vi "Loop_Vision.vi"() -> ()   [LabVIEW 2017, in "VisionSystem.lvlib"]
uses:
  VisionSystem.lvlib
  ENUM_Vision_State.ctl
  ENUM_Vision_Action.ctl
  Cluster_Results.ctl
  Cluster_Targeting Data.ctl
  Cluster_SGL Point.ctl
  Cluster_UI DBL Box.ctl
  Cluster_Vision Status.ctl
  Enum_ Field Targets.ctl
  Cluster_HW_Status.ctl
  <vilib>/vision/Image Controls.llb/IMAQ Image.ctl
  TypeDefs/Cluster_Camera Settings.ctl
  <vilib>/Rock Robotics/WPI/Camera/WPI_CameraImageSize.ctl
  <vilib>/Rock Robotics/WPI/Camera/WPI_CameraFrameRate.ctl
  <vilib>/Rock Robotics/WPI/Camera/WPI_CameraWhite Balance Values.ctl
  <vilib>/Rock Robotics/WPI/Camera/WPI_CameraExposure Values.ctl
  <vilib>/Rock Robotics/WPI/Camera/WPI_CameraDevRef.ctl
  Cluster_Vision Settings.ctl
  Cluster_Threshold Settings.ctl
  Cluster_Line.ctl
  ENUM_Camera Types.ctl
  _SHARE ALL/Global Share All/Global_STOP.vi
  Global_HW Status.vi
  Global_Vision Status.vi
panel:
  in  "Tab":enum32{"Boiler Settings", "Peg Settings"}(tab)
  in  "Boiler Setting":T1={"Color"={"Hue"={230.0, 10.0}, "Sat"={60.71428571428572, 255.0}, "Val"={63.75000000000001, 215.53571428571428}}, "Particles"=10.0, "Score Cutoff"=50.0, "Line Border"={"Top"=6.0, "Bottom"=1.0}, "Size Limit %"=0.04} {"Color"."Hue" scale=0.0..255.0 scale format="%#_3g"}
  in  "Peg Settings":T1={"Color"={"Hue"={235.0, 13.0}, "Sat"={0.0, 255.0}, "Val"={88.03571428571429, 221.60714285714286}}, "Particles"=10.0, "Score Cutoff"=50.0, "Line Border"={"Top"=6.0, "Bottom"=1.0}, "Size Limit %"=0.04} {"Color"."Hue" scale=0.0..255.0 scale format="%#_3g"}
  in  "Show Images":bool
  out "Errors":errorcluster[](array[cluster])
  out "HW_Vison_Status":T3 {"Cam Setings"."Saturation" min=0 max=100 step=1; "Cam Setings"."Sharpness" min=0 max=100 step=1; "Cam Setings"."Brightness" min=0 max=100 step=1; "Cam Setings"."Exposure (%)" min=0.0 max=100.0 step=1.0}
  out "Target":T10
  in  "Restore Settings":bool
  in  "Save Settings":bool
  out "Qualified Particles":i32
  out "Vision Status":T12
  out "Results":T13 {"Score" format="%#_3g"; "Pixels"."Box"."Bottom" format="%#_3g"; "Pixels"."Box"."Right" format="%#_3g"; "Pixels"."Box"."Top" format="%#_3g"; "Pixels"."Box"."Left" format="%#_3g"; "Normalized"."Box"."Bottom" format="%#_3g"; "Normalized"."Box"."Right" format="%#_3g"; "Normalized"."Box"."Top" format="%#_3g"; "Normalized"."Box"."Left" format="%#_3g"; "Distance (ft)" format="%#_3g"}
  out "cycle time":dbl
  out "Camera":T4(plugin-control)
  out "Mask":T4(plugin-control)
  out "Action":T17
  out "Current State":T18
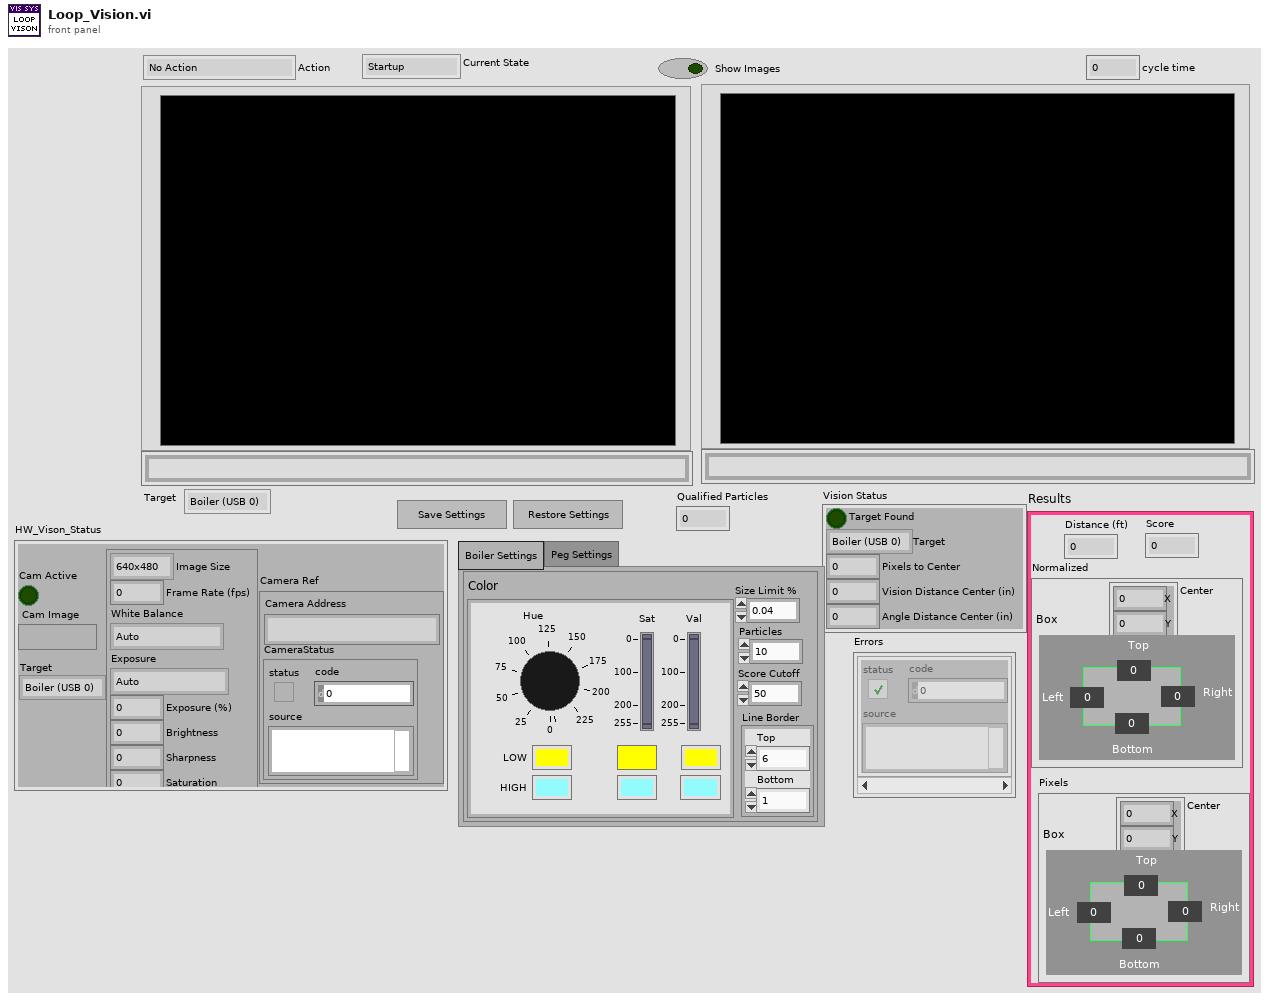
[diagram p1: front panel]
types:
  T1 = typedef "VisionSystem.lvlib/Cluster_Vision Settings.ctl" = cluster{"Color":T2, "Particles":dbl, "Score Cutoff":dbl, "Line Border":cluster{"Top":dbl, "Bottom":dbl}, "Size Limit %":dbl}
  T2 = typedef "VisionSystem.lvlib/Cluster_Threshold Settings.ctl" = cluster{"Hue":cluster{dbl, dbl}, "Sat":cluster{dbl, dbl}, "Val":cluster{dbl, dbl}}
  T3 = typedef "VisionSystem.lvlib/Cluster_HW_Status.ctl" = cluster{"Cam Active":bool, "Cam Image":T4, "Cam Setings":T5, "Target":T10, "Camera Ref":T11}
  T4 = typedef "IMAQ Image.ctl" = refnum<image>
  T5 = typedef "Cluster_Camera Settings.ctl" = cluster{"Image Size":T6, "Frame Rate (fps)":T7, "White Balance":T8, "Exposure":T9, "Exposure (%)":dbl, "Brightness":i32, "Sharpness":i32, "Saturation":i32}
  T6 = typedef "WPI_CameraImageSize.ctl" = enum16{"640x480", "320x240", "160x120", "Custom"}
  T7 = typedef "WPI_CameraFrameRate.ctl" = u32
  T8 = typedef "WPI_CameraWhite Balance Values.ctl" = enum16{"Auto", "Fixed indoor", "Fixed outdoor 1", "Fixed outdoor 2", "Fixed fluorescent 1", "Fixed fluorescent 2", "Hold current", "Custom"}
  T9 = typedef "WPI_CameraExposure Values.ctl" = enum16{"Auto", "Flicker-free 50 Hz", "Flicker-free 60 Hz", "Hold current", "Custom"}
  T10 = typedef "VisionSystem.lvlib/Enum_ Field Targets.ctl" = enum16{"Boiler (USB 0)", "Rope (USB 1)"}
  T11 = typedef "WPI_CameraDevRef.ctl" = cluster{"Camera Address":string, "CameraStatus":errorcluster}
  T12 = typedef "VisionSystem.lvlib/Cluster_Vision Status.ctl" = cluster{"Target Found":bool, "Target":T10, "Pixels to Center":dbl, "Vision Distance Center (in)":dbl, "Angle Distance Center (in)":dbl}
  T13 = typedef "VisionSystem.lvlib/Cluster_Results.ctl" = cluster{"Distance (ft)":dbl, "Score":dbl, "Normalized":T14, "Pixels":T14}
  T14 = typedef "VisionSystem.lvlib/Cluster_Targeting Data.ctl" = cluster{"Center":T15, "Box":T16}
  T15 = typedef "VisionSystem.lvlib/Cluster_SGL Point.ctl" = cluster{"X":sgl, "Y":sgl}
  T16 = typedef "VisionSystem.lvlib/Cluster_UI DBL Box.ctl" = cluster{"Left":dbl, "Top":dbl, "Right":dbl, "Bottom":dbl}
  T17 = typedef "VisionSystem.lvlib/ENUM_Vision_Action.ctl" = enum16{"No Action", "Reset Time", "Open Mask", "Close Mask", "Save Settings to File", "Restore Settings from File", "Build Mask", "Analyze Particles", "Cull and Group", "Calculate Distance", "Build Results", "Label Image"}
  T18 = typedef "VisionSystem.lvlib/ENUM_Vision_State.ctl" = enum16{"Startup", "Idle", "Analyze", "Shutdown"}
  T19 = typedef "VisionSystem.lvlib/Cluster_Line.ctl" = cluster{"Left":dbl, "Top":dbl, "Right":dbl, "Bottom":dbl}
  T20 = typedef "Particle Parameters" = i32
  T21 = cluster{"Actions":T17[], "State":T18, "Current Time":timestamp, "Start Time":timestamp, "Loop Time (ms)":u32, "HW_Status":T3, "Vision Status_OUT":T12, "Tab":enum32{"Boiler Settings", "Peg Settings"}, "Peg Settings":T1, "Boiler Settings":T1, "Mask":T4, "Measure List":T20[], "Current Settings":T1, "Show Images":bool, "Sorted Data":dbl[][], "Particles":i32, "Image":T4, "Center Out":T15, "Score Out":dbl, "Line Out":T19, "Rect Out":T16, "Distance (ft)":dbl, "Edges":T15[], "Results Out":T13, "Actions List":T17[]}
  T22 = typedef "VisionSystem.lvlib/ENUM_Camera Types.ctl" = enum16{"206", "1011", "1013", "MS HD3000 square", "MS HD3000 640x480"}
  T23 = typedef "Image Type" = u32
  T24 = typedef "VisionSystem.lvlib/Cluster_DBL Point.ctl" = cluster{"X":dbl, "Y":dbl}
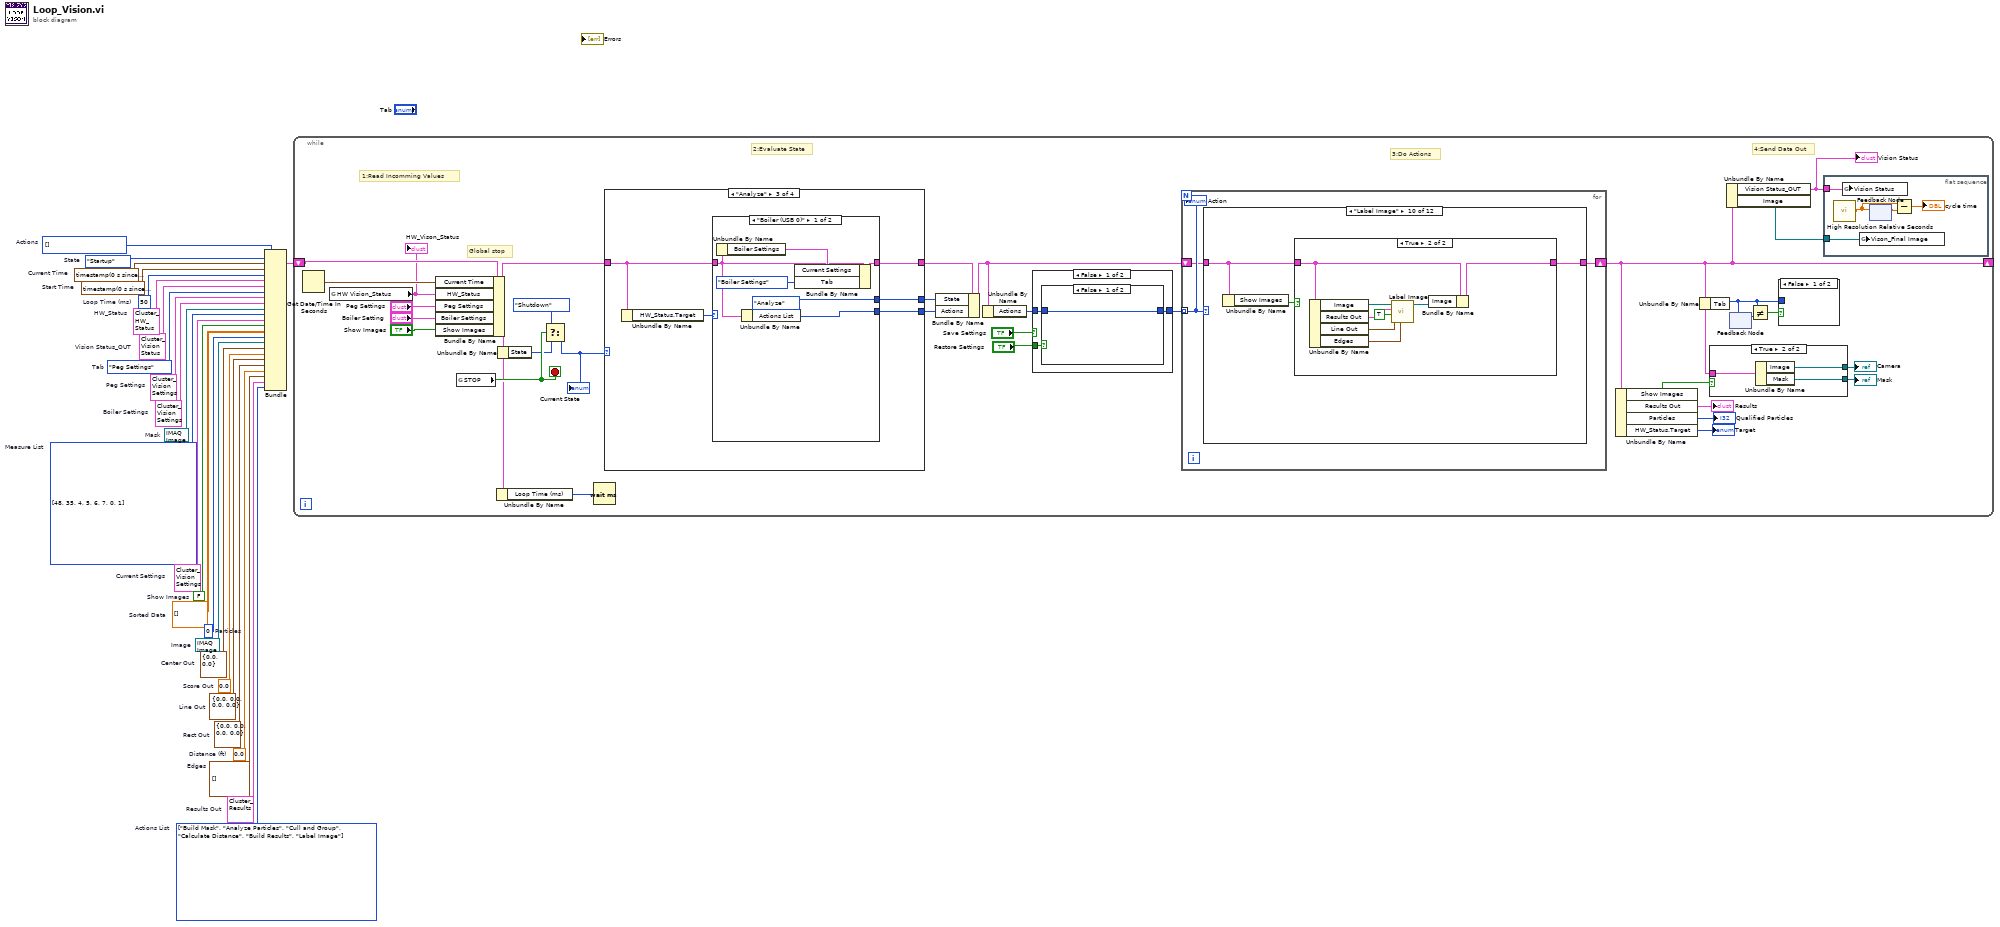
[diagram p0: block diagram]
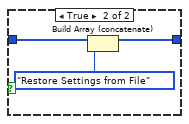
[diagram p2: hidden frame]
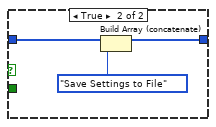
[diagram p3: hidden frame]
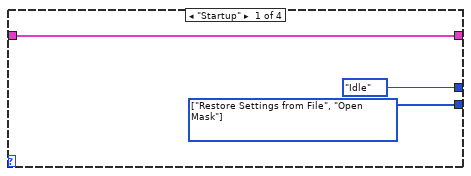
[diagram p4: hidden frame]
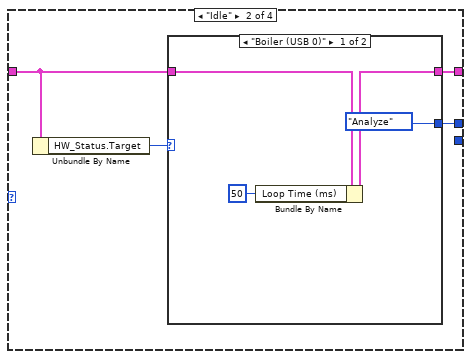
[diagram p5: hidden frame]
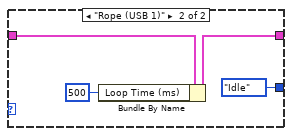
[diagram p6: hidden frame]
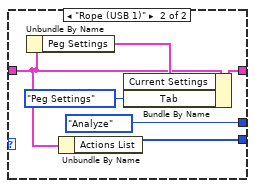
[diagram p7: hidden frame]
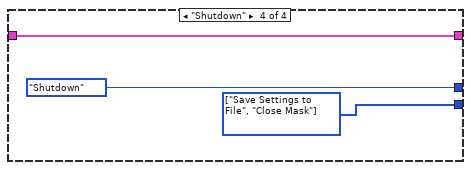
[diagram p8: hidden frame]
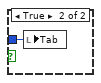
[diagram p10: hidden frame]
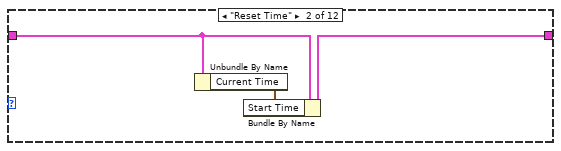
[diagram p12: hidden frame]
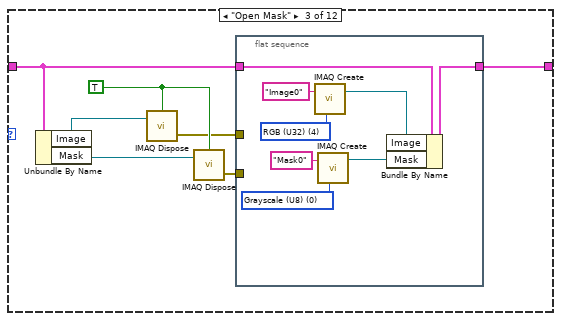
[diagram p13: hidden frame]
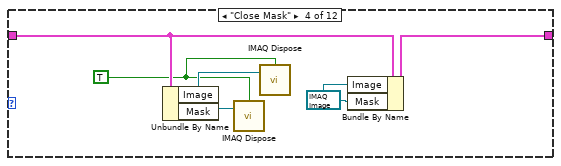
[diagram p14: hidden frame]
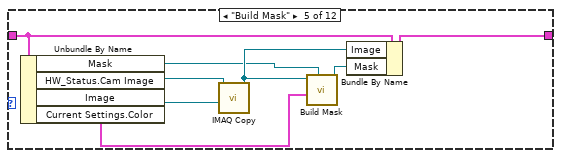
[diagram p15: hidden frame]
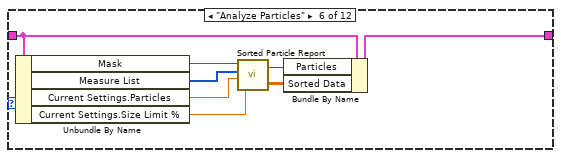
[diagram p16: hidden frame]
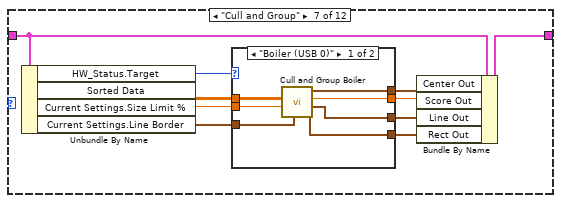
[diagram p17: hidden frame]
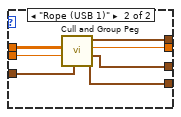
[diagram p18: hidden frame]
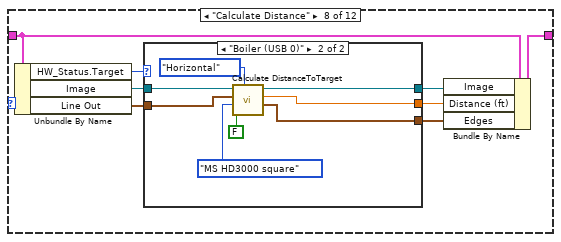
[diagram p19: hidden frame]
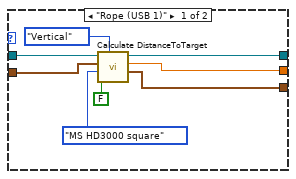
[diagram p20: hidden frame]
diagram:
  w1 = T17[] [enum."Build Mask", enum."Analyze Particles", enum."Cull and Group", enum."Calculate Distance", enum."Build Results", enum."Label Image"] items=["No Action", "Reset Time", "Open Mask", "Close Mask", "Save Settings to File", "Restore Settings from File", "Build Mask", "Analyze Particles", "Cull and Group", "Calculate Distance", "Build Results", "Label Image"]  # Actions List
  w2 = T13 {"Distance (ft)"=0.0, "Score"=0.0, "Normalized"={"Center"={"X"=0.0, "Y"=0.0}, "Box"={"Left"=0.0, "Top"=0.0, "Right"=0.0, "Bottom"=0.0}}, "Pixels"={"Center"={"X"=0.0, "Y"=0.0}, "Box"={"Left"=0.0, "Top"=0.0, "Right"=0.0, "Bottom"=0.0}}}  # Results Out
  w3 = T15[] []  # Edges
  w4 = 0.0  # Distance (ft)
  w5 = T16 {"Left"=0.0, "Top"=0.0, "Right"=0.0, "Bottom"=0.0}  # Rect Out
  w6 = T19 {"Left"=0.0, "Top"=0.0, "Right"=0.0, "Bottom"=0.0}  # Line Out
  w7 = 0.0  # Score Out
  w8 = T15 {"X"=0.0, "Y"=0.0}  # Center Out
  w9 = T4 refnum  # Image
  w10 = 0  # Particles
  w11 = dbl[][] []  # Sorted Data
  w12 = FALSE  # Show Images
  w13 = T1 {"Color"={"Hue"={235.0, 13.0}, "Sat"={97.0, 224.64285714285714}, "Val"={170.0, 255.0}}, "Particles"=10.0, "Score Cutoff"=50.0, "Line Border"={"Top"=6.0, "Bottom"=1.0}, "Size Limit %"=0.04}  # Current Settings
  w14 = T20[] [48, 35, 4, 5, 6, 7, 0, 1] items=["Center of Mass X", "Center of Mass Y", "First Pixel X", "First Pixel Y", "Bounding Rect Left", "Bounding Rect Top", "Bounding Rect Right", "Bounding Rect Bottom", "Max Feret Diameter Start X", "Max Feret Diameter Start Y", "Max Feret Diameter End X", "Max Feret Diameter End Y", "Max Horiz. Segment Length Left", "Max Horiz. Segment Length Right", "Max Horiz. Segment Length Row", "-", "Bounding Rect Width", "Bounding Rect Height", "Bounding Rect Diagonal", "Perimeter", "Convex Hull Perimeter", "Holes' Perimeter", "Max Feret Diameter", "Equivalent Ellipse Major Axis", "Equivalent Ellipse Minor Axis", "Equivalent Ellipse Minor Axis (Feret)", "Equivalent Rect Long Side", "Equivalent Rect Short Side", "Equivalent Rect Diagonal", "Equivalent Rect Short Side (Feret)", "Average Horiz. Segment Length", "Average Vert. Segment Length", "Hydraulic Radius", "Waddel Disk Diameter", "-", "Area", "Holes' Area", "Particle & Holes' Area", "Convex Hull Area", "Image Area", "-", "Number of Holes", "Number of Horiz. Segments", "Number of Vert. Segments", "-", "Orientation", "Max Feret Diameter Orientation", "-", "% Area/Image Area", "% Area/(Particle & Holes' Area)", "Ratio of Equivalent Ellipse Axes", "Ratio of Equivalent Rect Sides", "-", "Elongation Factor", "Compactness Factor", "Heywood Circularity Factor", "Type Factor", "-", "Sum X", "Sum Y", "Sum XX", "Sum XY", "Sum YY", "Sum XXX", "Sum XXY", "Sum XYY", "Sum YYY", "-", "Moment of Inertia XX", "Moment of Inertia XY", "Moment of Inertia YY", "Moment of Inertia XXX", "Moment of Inertia XXY", "Moment of Inertia XYY", "Moment of Inertia YYY", "Norm. Moment of Inertia XX", "Norm. Moment of Inertia XY", "Norm. Moment of Inertia YY", "Norm. Moment of Inertia XXX", "Norm. Moment of Inertia XXY", "Norm. Moment of Inertia XYY", "Norm. Moment of Inertia YYY", "Hu Moment 1", "Hu Moment 2", "Hu Moment 3", "Hu Moment 4", "Hu Moment 5", "Hu Moment 6", "Hu Moment 7"]  # Measure List
  w15 = T4 refnum  # Mask
  w16 = T1 {"Color"={"Hue"={235.0, 13.0}, "Sat"={97.0, 224.64285714285714}, "Val"={170.0, 255.0}}, "Particles"=10.0, "Score Cutoff"=50.0, "Line Border"={"Top"=6.0, "Bottom"=1.0}, "Size Limit %"=0.04}  # Boiler Settings
  w17 = T1 {"Color"={"Hue"={235.0, 13.0}, "Sat"={97.0, 224.64285714285714}, "Val"={170.0, 255.0}}, "Particles"=10.0, "Score Cutoff"=50.0, "Line Border"={"Top"=6.0, "Bottom"=1.0}, "Size Limit %"=0.04}  # Peg Settings
  w18 = enum32{"Boiler Settings", "Peg Settings"}."Peg Settings"  # Tab
  w19 = T12 {"Target Found"=FALSE, "Target"=enum."Boiler (USB 0)", "Pixels to Center"=0.0, "Vision Distance Center (in)"=0.0, "Angle Distance Center (in)"=0.0}  # Vision Status_OUT
  w20 = T3 {"Cam Active"=FALSE, "Cam Image"=refnum, "Cam Setings"={"Image Size"=enum."640x480", "Frame Rate (fps)"=0, "White Balance"=enum."Auto", "Exposure"=enum."Auto", "Exposure (%)"=0.0, "Brightness"=0, "Sharpness"=0, "Saturation"=0}, "Target"=enum."Boiler (USB 0)", "Camera Ref"={"Camera Address"="", "CameraStatus"={"status"=FALSE, "code"=0, "source"=""}}}  # HW_Status
  w21 = u32 50  # Loop Time (ms)
  w22 = T17[] [] items=["No Action", "Reset Time", "Open Mask", "Close Mask", "Save Settings to File", "Restore Settings from File", "Build Mask", "Analyze Particles", "Cull and Group", "Calculate Distance", "Build Results", "Label Image"]  # Actions
  w23 = timestamp(0 s since 1904-01-01)  # Start Time
  w24 = timestamp(0 s since 1904-01-01)  # Current Time
  w25 = ENUM_Vision_State."Startup"  # State
  n1 = Bundle("Actions"=w22, "State"=w25, "Current Time"=w24, "Start Time"=w23, "Loop Time (ms)"=w21, "HW_Status"=w20, "Vision Status_OUT"=w19, "Tab"=w18, "Peg Settings"=w17, "Boiler Settings"=w16, "Mask"=w15, "Measure List"=w14, "Current Settings"=w13, "Show Images"=w12, "Sorted Data"=w11, "Particles"=w10, "Image"=w9, "Center Out"=w8, "Score Out"=w7, "Line Out"=w6, "Rect Out"=w5, "Distance (ft)"=w4, "Edges"=w3, "Results Out"=w2, "Actions List"=w1) -> (w26:T21)  [unwired: 1 in]
  n2 = while {
    shift-right: [w32] -> _
    shift-left: w26 -> [w58]
    stop <- w53 stop-if-true
    # "1:Read Incomming Values"
    # "2:Evaluate State"
    # "3:Do Actions"
    # "4:Send Data Out"
    # "Global stop"
    n3 = Get Date/Time In Seconds() -> (seconds since 1Jan1904=w57:timestamp)
    n4 = global read "Global_HW Status.vi" "HW Vision_Status"() -> (w39:T3)
    "HW_Vison_Status" <- w39
    n5 = Bundle By Name(cluster=w58, "Current Time"=w57, "HW_Status"=w39, "Peg Settings"="Peg Settings", "Boiler Settings"="Boiler Setting", "Show Images"="Show Images") -> (w48:T21)
    n6 = global read "Global_STOP.vi" "STOP"() -> (w53:bool)
    n7 = Unbundle By Name(w48) -> ("Loop Time (ms)"=w49:u32)
    n8 = Unbundle By Name(w48) -> ("State"=w51:T18)
    n9 = Select(t=ENUM_Vision_State."Shutdown" ("State"), s=w53, f=w51) -> (s? t:f=w50:T18)
    "Current State" <- w50
    n10 = Wait (ms)(milliseconds to wait=w49) -> ()  [unwired: 1 out]
    n11 = case shown="\"Analyze\"" w50 {
      tunnel: w48 -> [w76 w79 w92 w108]
      tunnel: [w76 w78 w91 w108] -> w56
      tunnel: [ENUM_Vision_State."Idle" ("State") w77 w90 ENUM_Vision_State."Shutdown" ("State")] -> w55
      tunnel: [w75 _ w89 w106] -> w54
      frame "Startup" {
        w75 = T17[] [enum."Restore Settings from File", enum."Open Mask"] items=["No Action", "Reset Time", "Open Mask", "Close Mask", "Save Settings to File", "Restore Settings from File", "Build Mask", "Analyze Particles", "Cull and Group", "Calculate Distance", "Build Results", "Label Image"] ("Actions")
      }
      frame "Idle" {
        n12 = Unbundle By Name(w79) -> ("HW_Status.Target"=w80:T10)
        n13 = case shown="\"Boiler (USB 0)\"" w80 {
          tunnel: w79 -> [w83 w87]
          tunnel: [w82 w86] -> w78
          tunnel: [ENUM_Vision_State."Analyze" ("State") ENUM_Vision_State."Idle" ("State")] -> w77
          frame "Boiler (USB 0)" {
            n14 = Bundle By Name(cluster=w83, "Loop Time (ms)"=u32 50) -> (w82:T21)
          }
          frame "Rope (USB 1)" {
            n15 = Bundle By Name(cluster=w87, "Loop Time (ms)"=u32 500) -> (w86:T21)
          }
        }
      }
      frame "Analyze" {
        n16 = Unbundle By Name(w92) -> ("HW_Status.Target"=w93:T10)
        n17 = case shown="\"Boiler (USB 0)\"" w93 {
          tunnel: w92 -> [w95 w101]
          tunnel: [w98 w104] -> w91
          tunnel: [ENUM_Vision_State."Analyze" ("State") ENUM_Vision_State."Analyze" ("State")] -> w90
          tunnel: [w94 w100] -> w89
          frame "Boiler (USB 0)" {
            n18 = Unbundle By Name(w95) -> ("Boiler Settings"=w96:T1)
            n19 = Unbundle By Name(w95) -> ("Actions List"=w94:T17[])
            n20 = Bundle By Name(cluster=w95, "Current Settings"=w96, "Tab"=enum32{"Boiler Settings", "Peg Settings"}."Boiler Settings") -> (w98:T21)
          }
          frame "Rope (USB 1)" {
            n21 = Unbundle By Name(w101) -> ("Peg Settings"=w102:T1)
            n22 = Unbundle By Name(w101) -> ("Actions List"=w100:T17[])
            n23 = Bundle By Name(cluster=w101, "Current Settings"=w102, "Tab"=enum32{"Boiler Settings", "Peg Settings"}."Peg Settings") -> (w104:T21)
          }
        }
      }
      frame "Shutdown" {
        w106 = T17[] [enum."Save Settings to File", enum."Close Mask"] items=["No Action", "Reset Time", "Open Mask", "Close Mask", "Save Settings to File", "Restore Settings from File", "Build Mask", "Analyze Particles", "Cull and Group", "Calculate Distance", "Build Results", "Label Image"] ("Actions")
      }
    }
    n24 = Bundle By Name(cluster=w56, "State"=w55, "Actions"=w54) -> (w34:T21)
    n25 = Unbundle By Name(w34) -> ("Actions"=w36:T17[])
    n26 = case shown="False" "Save Settings" {
      tunnel: "Restore Settings" -> [w61 _]
      tunnel: w36 -> [w60 w67]
      tunnel: [w59 w66] -> w35
      frame False {
        n27 = case shown="False" w61 {
          tunnel: w60 -> [w62 w65]
          tunnel: [w62 w64] -> w59
          frame False {
          }
          frame True {
            n28 = Build Array (concatenate)(w65, ENUM_Vision_Action."Restore Settings from File" ("Action 2")) -> (w64:T17[])
          }
        }
      }
      frame True {
        n29 = Build Array (concatenate)(w67, ENUM_Vision_Action."Save Settings to File" ("Action 2")) -> (w66:T17[])
      }
    }
    n30 = for {
      tunnel: w35 -> [w115] mode=indexing
      shift-right: [w114] -> w32
      shift-left: w34 -> [w113]
      n31 = case shown="\"Label Image\"" w115 {
        tunnel: w113 -> [w116 w119 w125 w139 w148 w152 w165 w182 w211 w219 w235 w240]
        tunnel: [w116 w118 w126 w140 w147 w151 w166 w181 w210 w218 w235 w239] -> w114
        frame "No Action" {
        }
        frame "Reset Time" {
          n32 = Unbundle By Name(w119) -> ("Current Time"=w117:timestamp)
          n33 = Bundle By Name(cluster=w119, "Start Time"=w117) -> (w118:T21)
        }
        frame "Open Mask" {
          w121 = TRUE ("All Images? (No)")
          n34 = Unbundle By Name(w125) -> ("Image"=w122:T4, "Mask"=w124:T4)
          n35 = call "IMAQ Dispose"("All Images? (No)"=w121, "Image"=w122) -> ("error out"=w120:errorcluster)  [unwired: 4 in]
          n36 = call "IMAQ Dispose"("All Images? (No)"=w121, "Image"=w124) -> ("error out"=w123:errorcluster)  [unwired: 4 in]
          n37 = flat-sequence {
            tunnel: w125 -> [w134]
            tunnel: [w133] -> w126
            tunnel: w123 -> [_]
            tunnel: w120 -> [_]
            frame #0 {
              w129 = T23 4 items=["Grayscale (U8)", "Grayscale (I16)", "Grayscale (SGL)", "Complex (CSG)", "RGB (U32)", "HSL (U32)", "RGB (U64)", "Grayscale (U16)"] ("Image Type")
              w131 = T23 0 items=["Grayscale (U8)", "Grayscale (I16)", "Grayscale (SGL)", "Complex (CSG)", "RGB (U32)", "HSL (U32)", "RGB (U64)", "Grayscale (U16)"] ("Image Type")
              n38 = call "IMAQ Create"("Image Name"="Image0", "Image Type"=w129) -> ("New Image"=w127:T4)  [unwired: 2 in, 2 out]
              n39 = call "IMAQ Create"("Image Name"="Mask0", "Image Type"=w131) -> ("New Image"=w130:T4)  [unwired: 2 in, 2 out]
              n40 = Bundle By Name(cluster=w134, "Image"=w127, "Mask"=w130) -> (w133:T21)
            }
          }
        }
        frame "Close Mask" {
          w137 = T4 refnum ("Mask")
          w135 = TRUE ("All Images? (No)")
          n41 = Unbundle By Name(w139) -> ("Image"=w136:T4, "Mask"=w138:T4)
          n42 = call "IMAQ Dispose"("All Images? (No)"=w135, "Image"=w138) -> ()  [unwired: 4 in, 1 out]
          n43 = call "IMAQ Dispose"("All Images? (No)"=w135, "Image"=w136) -> ()  [unwired: 4 in, 1 out]
          n44 = Bundle By Name(cluster=w139, "Image"=w137, "Mask"=w137) -> (w140:T21)
        }
        frame "Build Mask" {
          n45 = Unbundle By Name(w148) -> ("Mask"=w141:T4, "HW_Status.Cam Image"=w143:T4, "Image"=w144:T4, "Current Settings.Color"=w145:T2)
          n46 = call "IMAQ Copy"("Image Dst"=w144, "Image Src"=w143) -> ("Image Dst Out"=w142:T4)  [unwired: 4 in, 1 out]
          n47 = call "Build Mask.vi"("Mask"=w141, "Color"=w145, "Cam Image"=w142) -> ("Mask Out"=w146:T4)  [unwired: 7 in, 1 out]
          n48 = Bundle By Name(cluster=w148, "Image"=w142, "Mask"=w146) -> (w147:T21)
        }
        frame "Analyze Particles" {
          n49 = Unbundle By Name(w152) -> ("Mask"=w156:T4, "Measure List"=w155:T20[], "Current Settings.Particles"=w154:dbl, "Current Settings.Size Limit %"=w153:dbl)
          n50 = call "Sorted Particle Report.vi"("Min Area Size %"=w153, "Particle Count Limit"=w154, "Pixel Measurements"=w155, "Image in"=w156) -> ("Sorted Data"=w150:dbl[][], "Particles"=w149:i32)
          n51 = Bundle By Name(cluster=w152, "Particles"=w149, "Sorted Data"=w150) -> (w151:T21)
        }
        frame "Cull and Group" {
          n52 = Unbundle By Name(w165) -> ("HW_Status.Target"=w157:T10, "Sorted Data"=w164:dbl[][], "Current Settings.Size Limit %"=w163:dbl, "Current Settings.Line Border"=w162:cluster{"Top":dbl, "Bottom":dbl})
          n53 = case shown="\"Boiler (USB 0)\"" w157 {
            tunnel: w164 -> [w173 w180]
            tunnel: w163 -> [w172 w179]
            tunnel: w162 -> [w171 w178]
            tunnel: [w170 w177] -> w161
            tunnel: [w169 w176] -> w160
            tunnel: [w168 w174] -> w159
            tunnel: [w167 w175] -> w158
            frame "Boiler (USB 0)" {
              n54 = call "Cull and Group Boiler.vi"("Line Border"=w171, "Score Cutoff"=w172, "Sorted Data"=w173) -> ("Rect Out"=w167:T16, "Line Out"=w168:T19, "Score Out"=w169:dbl, "Center Out"=w170:T15)  [unwired: 5 in]
            }
            frame "Rope (USB 1)" {
              n55 = call "Cull and Group Peg.vi"("Line Border"=w178, "Score Cutoff"=w179, "Sorted Data"=w180) -> ("Rect Out"=w175:T16, "Line Out"=w174:T19, "Top Score Out"=w176:dbl, "Center Out"=w177:T24)  [unwired: 5 in]
            }
          }
          n56 = Bundle By Name(cluster=w165, "Center Out"=w161, "Score Out"=w160, "Line Out"=w159, "Rect Out"=w158) -> (w166:T21)
        }
        frame "Calculate Distance" {
          n57 = Unbundle By Name(w182) -> ("HW_Status.Target"=w186:T10, "Image"=w188:T4, "Line Out"=w187:T19)
          n58 = case shown="\"Boiler (USB 0)\"" w186 {
            tunnel: w188 -> [w196 w204]
            tunnel: w187 -> [w194 w202]
            tunnel: [w191 w199] -> w185
            tunnel: [w190 w198] -> w184
            tunnel: [w189 w197] -> w183
            frame "Rope (USB 1)" {
              n59 = call "Calculate DistanceToTarget.vi"("Type"=enum16{"Horizontal", "Vertical", "Diagonal"}."Vertical", "Calibrated"=FALSE, "Camera Type"=ENUM_Camera_Types."MS HD3000 square", "Line"=w194, "Image Src"=w196) -> ("Edges"=w189:T15[], "Distance (ft)"=w190:dbl, "Image Dst Out"=w191:T4)  [unwired: 4 in]
            }
            frame "Boiler (USB 0)" {
              n60 = call "Calculate DistanceToTarget.vi"("Type"=enum16{"Horizontal", "Vertical", "Diagonal"}."Horizontal", "Calibrated"=FALSE, "Camera Type"=ENUM_Camera_Types."MS HD3000 square", "Line"=w202, "Image Src"=w204) -> ("Edges"=w197:T15[], "Distance (ft)"=w198:dbl, "Image Dst Out"=w199:T4)  [unwired: 4 in]
            }
          }
          n61 = Bundle By Name(cluster=w182, "Image"=w185, "Distance (ft)"=w184, "Edges"=w183) -> (w181:T21)
        }
        frame "Build Results" {
          n62 = Unbundle By Name(w211) -> ("Image"=w216:T4, "Rect Out"=w215:T16, "Distance (ft)"=w214:dbl, "Center Out"=w213:T15, "Score Out"=w212:dbl, "HW_Status.Target"=w207:T10, "HW_Status.Cam Setings.Image Size"=w206:T6)
          n63 = call "Build Results.vi"("Score"=w212, "Center"=w213, "Distance"=w214, "Bounding Box"=w215, "Image"=w216) -> ("Results Out"=w208:T13, "Image Out"=w209:T4)  [unwired: 5 in]
          n64 = call "Build Global Data.vi"("Target"=w207, "Image Size"=w206, "Results"=w208) -> ("Vision Data Out"=w205:T12)  [unwired: 8 in]
          n65 = Bundle By Name(cluster=w211, "Image"=w209, "Results Out"=w208, "Vision Status_OUT"=w205) -> (w210:T21)
        }
        frame "Label Image" {
          n66 = Unbundle By Name(w219) -> ("Show Images"=w217:bool)
          n67 = case shown="True" w217 {
            tunnel: w219 -> [w220 w223]
            tunnel: [w220 w222] -> w218
            frame False {
            }
            frame True {
              n68 = Unbundle By Name(w223) -> ("Image"=w228:T4, "Results Out"=w227:T13, "Line Out"=w225:T19, "Edges"=w224:T15[])
              n69 = call "Label Image.vi"("Edges"=w224, "Line"=w225, "Annotate"=TRUE, "Results"=w227, "Image"=w228) -> ("Image Out"=w221:T4)  [unwired: 6 in]
              n70 = Bundle By Name(cluster=w223, "Image"=w221) -> (w222:T21)
            }
          }
        }
        frame "Save Settings to File" {
          n71 = Unbundle By Name(w235) -> ("Peg Settings"=w232:T1, "Boiler Settings"=w231:T1)
          n72 = call "Read-Write Vision Settings to File.vi"("Read(f)Write(t)"=TRUE, "Target"=Enum__Field_Targets."Boiler (USB 0)", "Vision Settings"=w231) -> ("Error Out"=w233:errorcluster)  [unwired: 6 in, 2 out]
          n73 = call "Read-Write Vision Settings to File.vi"("Read(f)Write(t)"=TRUE, "Target"=Enum__Field_Targets."Rope (USB 1)", "Error"=w233, "Vision Settings"=w232) -> ()  [unwired: 5 in, 3 out]
        }
        frame "Restore Settings from File" {
          n74 = call "Read-Write Vision Settings to File.vi"("Read(f)Write(t)"=FALSE, "Target"=Enum__Field_Targets."Boiler (USB 0)") -> ("Error Out"=w243:errorcluster, "Vision Settings Out"=w237:T1)  [unwired: 7 in, 1 out]
          n75 = call "Read-Write Vision Settings to File.vi"("Read(f)Write(t)"=FALSE, "Target"=Enum__Field_Targets."Rope (USB 1)", "Error"=w243) -> ("Vision Settings Out"=w238:T1)  [unwired: 6 in, 2 out]
          n76 = Bundle By Name(cluster=w240, "Peg Settings"=w238, "Boiler Settings"=w237) -> (w239:T21)
        }
      }
      "Action" <- w115
    }
    n77 = Unbundle By Name(w32) -> ("Show Images"=w31:bool, "Results Out"=→"Results":T13, "Particles"=→"Qualified Particles":i32, "HW_Status.Target"=→"Target":T10)
    n78 = Unbundle By Name(w32) -> ("Tab"=w44:enum32{"Boiler Settings", "Peg Settings"})
    n79 = case shown="True" w31 {
      tunnel: w32 -> [_ w111]
      tunnel: [_ w110] -> w41
      tunnel: [_ w109] -> w40
      frame False {
      }
      frame True {
        n80 = Unbundle By Name(w111) -> ("Image"=w110:T4, "Mask"=w109:T4)
      }
    }
    "Camera" <- w41
    "Mask" <- w40
    n81 = Unbundle By Name(w32) -> ("Vision Status_OUT"=w45:T12, "Image"=w27:T4)
    "Vision Status" <- w45
    n82 = feedback #1() -> (w47:enum32{"Boiler Settings", "Peg Settings"})  [unwired: 1 in]
    n83 = feedback-in #1(w44) -> ()
    n84 = Not Equal?(x=w44, y=w47) -> (x != y?=w46:bool)
    n85 = case shown="False" w46 {
      tunnel: w44 -> [_ w112]
      frame False {
      }
      frame True {
        n86 = local write "Tab"(w112) -> ()
      }
    }
    n87 = flat-sequence {
      tunnel: w45 -> [w73]
      tunnel: w27 -> [w69]
      frame #0 {
        n88 = call <vilib>:"High Resolution Relative Seconds.vi"() -> ("relative seconds"=w72:dbl)
        n89 = global write "Global_Vision Status.vi" "Vision Status"(w73) -> ()
        n90 = global write "Global_Vision Status.vi" "Vison_Final Image"(w69) -> ()
        n91 = feedback #2() -> (w71:dbl)  [unwired: 1 in]
        n92 = feedback-in #2(w72) -> ()
        n93 = Subtract(x=w72, y=w71) -> (x-y=→"cycle time":dbl)
      }
    }
  }
